vi "Renew Tools Control Position.vi"(8 "error in (no error)":errorcluster, 11 "ScriptDialog":refnum<class "ScriptDialog.lvclass">) -> (0 "error out":errorcluster, 3 "ScriptDialog  Out":refnum<class "ScriptDialog.lvclass">)   [LabVIEW 2015, in "ScriptDialog.lvclass"]
uses:
  ScriptDialog.lvclass
  ScriptDialog.lvclass/ScriptDialog.ctl
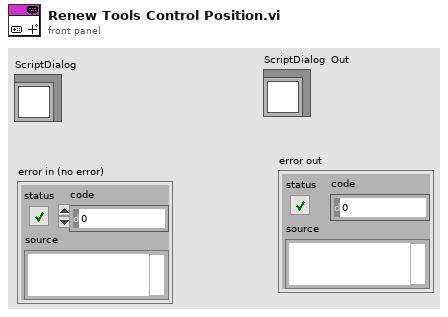
[diagram p1: front panel]
types:
  T1 = typedef "LVPositionTypeDef.ctl" = cluster{"Left":i32, "Top":i32}
  T2 = typedef "LVBoundsTypeDef.ctl" = cluster{"Width":u32, "Height":u32}
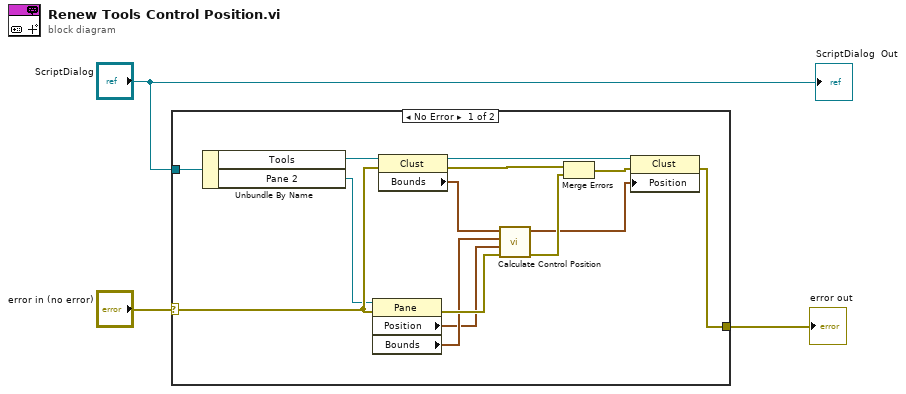
[diagram p0: block diagram]
diagram:
  n1 = case shown="No Error" "error in (no error)" {
    selector: "error in (no error)" -> [w11 w18]
    tunnel: "ScriptDialog" -> [w14 _]
    tunnel: [w5 w18] -> w1
    frame No Error {
      n2 = Unbundle By Name(w14) -> ("Tools"=w13:refnum<vi>, "Pane 2"=w4:refnum<vi>)
      n3 = property class="Pane"(reference=w4, error in=w11) -> (error out=w17:errorcluster, "Position"=w15:T1, "Bounds"=w16:T2)  [unwired: 1 out]
      n4 = property class="Clust"(reference=w13, error in=w11) -> (reference out=w10:refnum<vi>, error out=w9:errorcluster, "Bounds"=w12:T2)
      n5 = call "Calculate Control Position.vi"("error in (no error)"=w17, "Panel Position"=w15, "Panel Bound"=w16, "Control Bound"=w12) -> ("error out"=w8:errorcluster, "Control Position Out"=w6:T1)  [unwired: 6 in]
      n6 = Merge Errors(w9, w8) -> (w7:errorcluster)
      n7 = property class="Clust"(reference=w10, error in=w7, "Position"=w6) -> (error out=w5:errorcluster)  [unwired: 1 out]
    }
    frame Error {
    }
  }
  "error out" <- w1
  "ScriptDialog  Out" <- "ScriptDialog"
